vi "Move absolute.vi"(0 "Zaber":T1={"Serial port handle"="", "Axis"="", "Controller #"=0, "Min position"=0.0, "Max position"=0.0, "Min velocity"=0.0, "Max velocity"=0.0, "Firmware"="", "Device ID"=0, "Variable event"=refnum, "Variable ref"=refnum, "Resolution, usteps/step"=0, "Serial port semaphore"=refnum, "Joystick buttons"={"MinDir"=1, "MaxDir"=2, "MedSpeed"=5, "HighSpeed"=6}} {"Joystick buttons"."HighSpeed" min=1 max=25 step=1; "Joystick buttons"."MedSpeed" min=1 max=25 step=1; "Joystick buttons"."MaxDir" min=1 max=25 step=1; "Joystick buttons"."MinDir" min=1 max=25 step=1}, 2 "Position, mm":dbl, 5 "error in":errorcluster) -> (11 "Start time, ms":u32, 14 "Zaber out":T1={"Serial port handle"="", "Axis"="", "Controller #"=0, "Min position"=0.0, "Max position"=0.0, "Min velocity"=0.0, "Max velocity"=0.0, "Firmware"="", "Device ID"=0, "Variable event"=refnum, "Variable ref"=refnum, "Resolution, usteps/step"=0, "Serial port semaphore"=refnum, "Joystick buttons"={"MinDir"=1, "MaxDir"=2, "MedSpeed"=5, "HighSpeed"=6}} {"Joystick buttons"."HighSpeed" min=1 max=25 step=1; "Joystick buttons"."MedSpeed" min=1 max=25 step=1; "Joystick buttons"."MaxDir" min=1 max=25 step=1; "Joystick buttons"."MinDir" min=1 max=25 step=1}, 16 "Position, mm":dbl, 19 "error out":errorcluster)   [LabVIEW 2018]
uses:
  Zaber.ctl
  GenericDataEvent/GenericEvent.ctl
  ZaberVariables.ctl
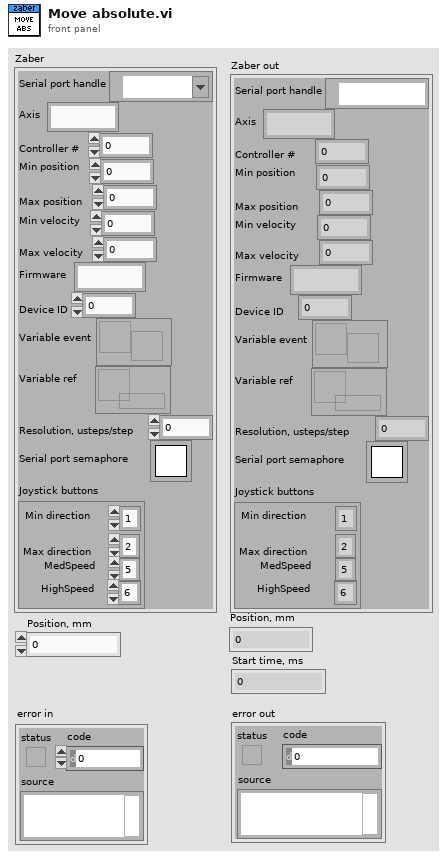
[diagram p1: front panel]
types:
  T1 = typedef "Zaber.ctl" = cluster{"Serial port handle":refnum<visa-resource-name>, "Axis":string, "Controller #":u8, "Min position":dbl, "Max position":dbl, "Min velocity":dbl, "Max velocity":dbl, "Firmware":string, "Device ID":i32, "Variable event":T2, "Variable ref":refnum<data-value>, "Resolution, usteps/step":i32, "Serial port semaphore":T3, "Joystick buttons":cluster{"MinDir":i32, "MaxDir":i32, "MedSpeed":i32, "HighSpeed":i32}}
  T2 = typedef "GenericEvent.ctl" = refnum<user-event>
  T3 = typedef "Semaphore RefNum" = refnum<k1>
  T4 = typedef "ZaberVariables.ctl" = cluster{"Position":i32, "Speed":i32, "Min soft position":dbl, "Max soft position":dbl, "Accelaration":i32}
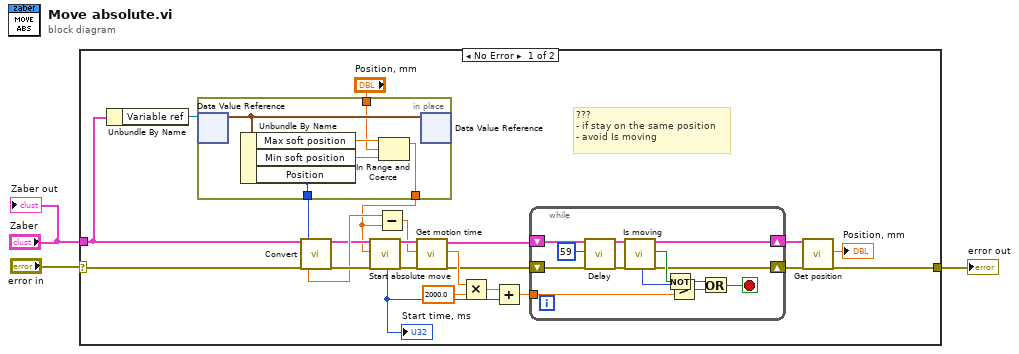
[diagram p0: block diagram]
diagram:
  n1 = case shown="No Error" "error in" {
    selector: "error in" -> [w6 w45]
    tunnel: [w20 w45] -> w2
    tunnel: "Zaber" -> [w8 _]
    frame No Error {
      # "???\n- if stay on the same position\n- avoid Is moving"
      n2 = Unbundle By Name(w8) -> ("Variable ref"=w12:refnum<data-value>)
      n3 = in-place {
        in-place-border: [w31] -> w10
        in-place-border: "Position, mm" -> [w28]
        in-place-border: [w27] -> w4
        n4 = in-place-dvr #1(w12) -> (w32:T4)  [unwired: 1 out]
        n5 = Unbundle By Name(w32) -> ("Max soft position"=w30:dbl, "Min soft position"=w29:dbl, "Position"=w31:i32)
        n6 = In Range and Coerce(upper limit=w30, x=w28, lower limit=w29) -> (coerced(x)=w27:dbl)  [unwired: 1 out]
        n7 = in-place-dvr #1(w32) -> ()  [unwired: 2 out]
      }
      n8 = call "Convert.vi"("Zaber"=w8, "error in"=w6, "Position, usteps"=w10) -> ("Position, mm"=w9:dbl, "Zaber out"=w7:T1, "error out"=w11:errorcluster)  [unwired: 8 in, 6 out]
      n9 = call "Start absolute move.vi"("Zaber"=w7, "Position, mm"=w4, "error in"=w11) -> ("Start time, ms"=w18:u32, "Zaber out"=w15:T1, "error out"=w25:errorcluster)  [unwired: 14 in]
      "Start time, ms" <- w18
      n10 = Subtract(x=w9, y=w4) -> (x-y=w14:dbl)
      n11 = call "Get motion time.vi"("Zaber"=w15, "Distance, mm"=w14, "error in"=w25) -> ("Zaber out"=w26:T1, "Motion time, s"=w17:dbl, "error out"=w16:errorcluster)  [unwired: 14 in]
      n12 = Multiply(x=w17, y=2000.0) -> (x*y=w22:dbl)
      n13 = Add(x=w22, y=w18) -> (x+y=w23:dbl)
      n14 = while {
        shift-right: [w34] -> w21
        shift-left: w16 -> [w41]
        tunnel: w23 -> [w44]
        shift-right: [w38] -> w13
        shift-left: w26 -> [w33]
        stop <- w42 stop-if-true
        n15 = call "Delay.vi"("Delay, ms"=u32 59, "error in"=w41) -> ("error out"=w40:errorcluster)  [unwired: 17 in]
        n16 = call "Is moving.vi"("Zaber"=w33, "error in"=w40) -> ("Command time, ms"=w35:u32, "Zaber out"=w38:T1, "Is moving?"=w37:bool, "error out"=w34:errorcluster)  [unwired: 14 in]
        n17 = Not(x=w37) -> (.not. x?=w36:bool)
        n18 = Greater?(x=w35, y=w44) -> (0:w43:bool)
        n19 = Or(x=w36, y=w43) -> (x .or. y?=w42:bool)
      }
      n20 = call "Get position.vi"("Zaber"=w13, "error in"=w21) -> ("PositionRb"=→"Position, mm":dbl, "error out"=w20:errorcluster)  [unwired: 13 in, 3 out]
    }
    frame Error {
    }
  }
  "error out" <- w2
  "Zaber out" <- "Zaber"
